vi "LVClass_WavefrontCorrectorSet Write WavefrontCorrectorSet.vi"(8 "error in (no error)":errorcluster, 10 "WavefrontCorrectorSet":T1, 11 "WavefrontCorrectorSet in":refnum<class "WavefrontCorrectorSet.lvclass">) -> (0 "error out":errorcluster, 3 "WavefrontCorrectorSet out":refnum<class "WavefrontCorrectorSet.lvclass">)   [LabVIEW 2020, in "WavefrontCorrectorSet.lvclass"]
uses:
  WavefrontCorrectorSet.lvclass
  Controls/ClassID.ctl
  Controls/Handle creation.ctl
  WavefrontCorrectorSet.lvclass/WavefrontCorrectorSet.ctl
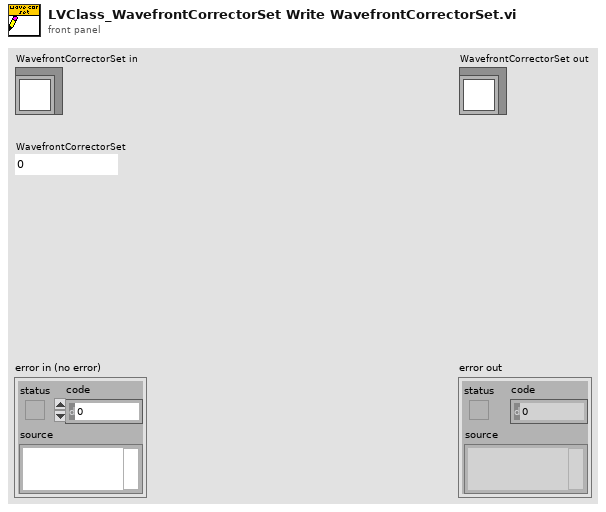
[diagram p1: front panel]
types:
  T1 = typedef "ClassID.ctl" = i64
  T2 = typedef "Handle creation.ctl" = enum16{"By ctor", "By write function"}
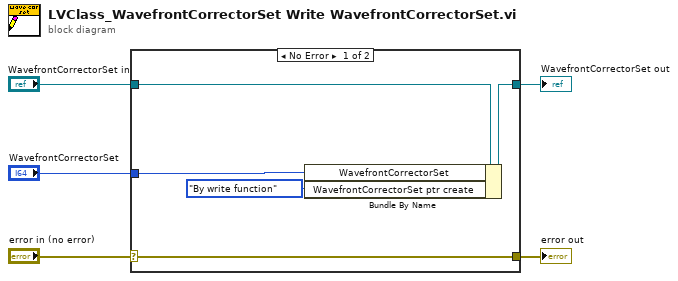
[diagram p0: block diagram]
diagram:
  n1 = case shown="No Error" "error in (no error)" {
    selector: "error in (no error)" -> [w10 w11]
    tunnel: [w10 w11] -> w4
    tunnel: [w8 w12] -> w2
    tunnel: "WavefrontCorrectorSet in" -> [w9 w12]
    tunnel: "WavefrontCorrectorSet" -> [w7 _]
    frame No Error {
      n2 = Bundle By Name(cluster=w9, "WavefrontCorrectorSet"=w7, "WavefrontCorrectorSet ptr create"=Handle_creation."By write function") -> (w8:refnum<class "WavefrontCorrectorSet.lvclass">)
    }
    frame Error {
    }
  }
  "error out" <- w4
  "WavefrontCorrectorSet out" <- w2
